vi "Shooter_Motor.vi"(0 "MotorControlDevRef":T2={"DeviceStatus"={"status"=FALSE, "code"=0, "source"=""}, "Type"=enum."PWM", "PWM"={"PWM Channel"=enum."Invalid", "DeadBand"={"Name"="", "maxPositivePwm"=0, "minPositivePwm"=0, "centerPwm"=0, "maxNegativePwm"=0, "minNegativePwm"=0, "angularRange"=0}}, "CAN"={"Device Number"=0, "SetOutput VI Ref"=variant(refnum<vi> refnum), "GetOutput VI Ref"=variant(refnum<vi> refnum), "Enable VI Ref"=variant(refnum<vi> refnum), "Disable VI Ref"=variant(refnum<vi> refnum), "Data"=variant}, "Invert"=FALSE}, 1 "Invert?":bool, 2 "RPM_Input":dbl, 3 "Wanted_RPM":dbl=1.0, 4 "dt_In_PID":dbl, 5 "PID gains":T1={"proportional gain (Kc)"=1.0, "integral time (Ti, min)"=0.01, "derivative time (Td, min)"=0.0} {"derivative time (Td, min)" format="%.3f"; "integral time (Ti, min)" format="%.3f"; "proportional gain (Kc)" format="%.3f"}) -> (14 "Shooter_Speed":dbl, 15 "dt_Out_PID":dbl, 16 "RPM_Reached?":bool)   [LabVIEW 2016]
uses:
  <vilib>/Rock Robotics/WPI/MotorControl/WPI_MotorControlDeviceRef.ctl
  <vilib>/Rock Robotics/WPI/MotorControl/WPI_MotorControlType.ctl
  <vilib>/Rock Robotics/SystemInterfaces/DIO/FPGA_DIOPWMChannel.ctl
  <vilib>/Rock Robotics/WPI/PWM/WPI_PWMDeadband.ctl
  <vilib>/addons/control/pid/pid.llb/PID (DBL).vi
  <vilib>/addons/control/pid/NI_PID_pid.lvlib
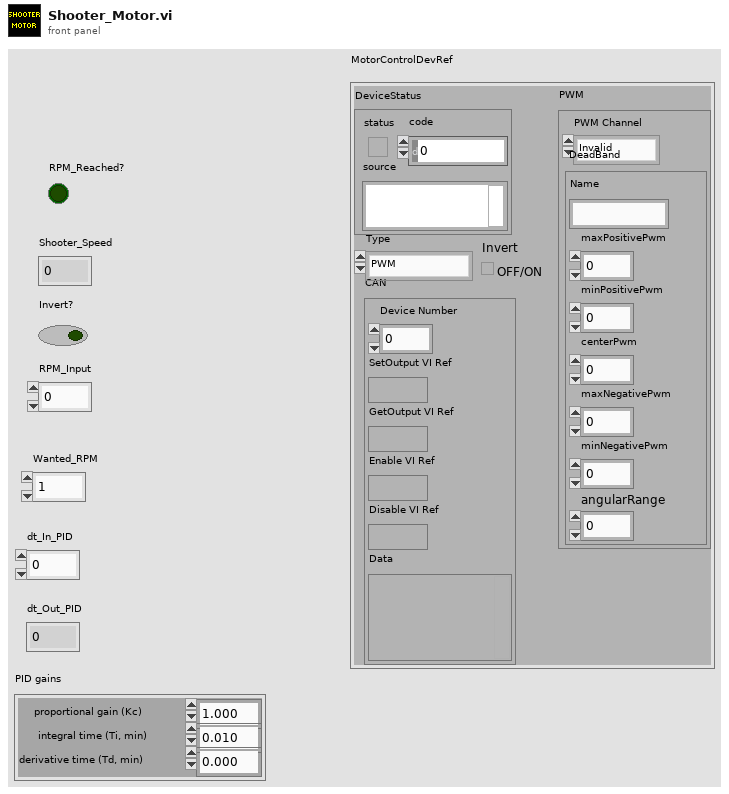
[diagram p1: front panel]
types:
  T1 = cluster{"proportional gain (Kc)":dbl, "integral time (Ti, min)":dbl, "derivative time (Td, min)":dbl}
  T2 = typedef "WPI_MotorControlDeviceRef.ctl" = cluster{"DeviceStatus":errorcluster, "Type":T3, "PWM":cluster{"PWM Channel":T4, "DeadBand":T5}, "CAN":cluster{"Device Number":u8, "SetOutput VI Ref":variant, "GetOutput VI Ref":variant, "Enable VI Ref":variant, "Disable VI Ref":variant, "Data":variant}, "Invert":bool}
  T3 = typedef "WPI_MotorControlType.ctl" = enum16{"PWM", "CAN"}
  T4 = typedef "FPGA_DIOPWMChannel.ctl" = enum8{"PWM 0", "PWM 1", "PWM 2", "PWM 3", "PWM 4", "PWM 5", "PWM 6", "PWM 7", "PWM 8", "PWM 9", "PWM MXP 0", "PWM MXP 1", "PWM MXP 2", "PWM MXP 3", "PWM MXP 4", "PWM MXP 5", "PWM MXP 6", "PWM MXP 7", "PWM MXP 8", "PWM MXP 9", "Invalid"}
  T5 = typedef "WPI_PWMDeadband.ctl" = cluster{"Name":string, "maxPositivePwm":i32, "minPositivePwm":i32, "centerPwm":i32, "maxNegativePwm":i32, "minNegativePwm":i32, "angularRange":u16}
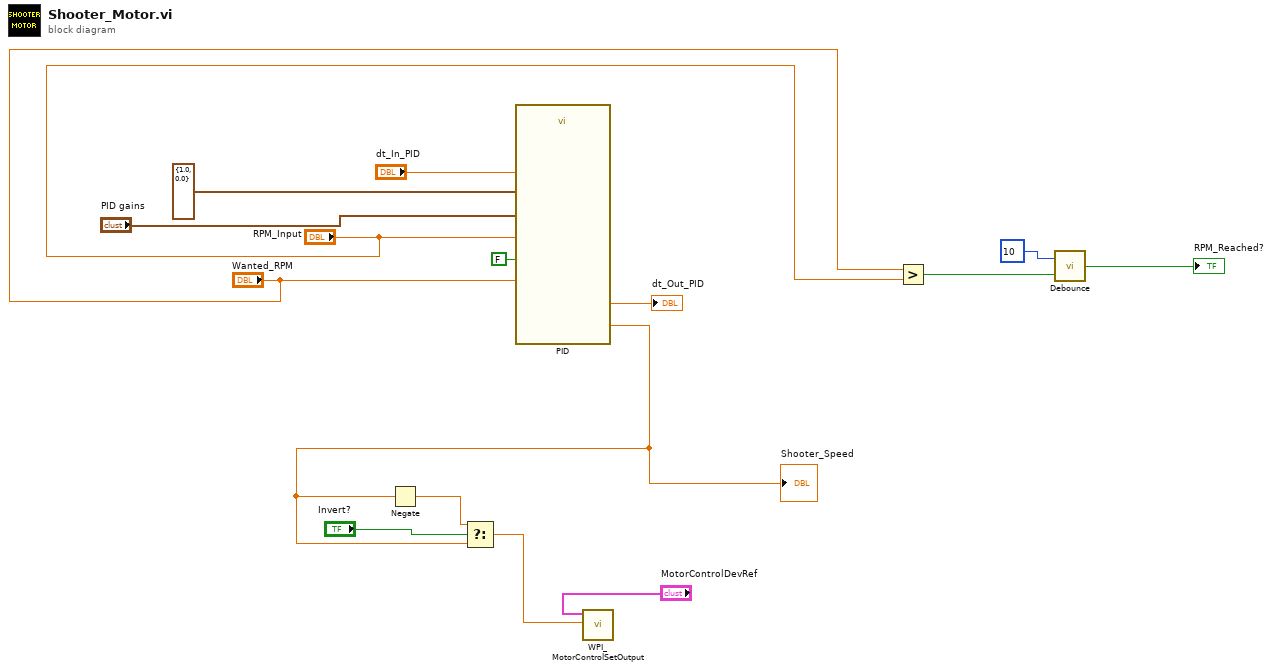
[diagram p0: block diagram]
diagram:
  n1 = call-poly <vilib>:"PID.vi"("reinitialize? (F)"=FALSE, "output range"=cluster{"output high":dbl, "output low":dbl} {"output high"=1.0, "output low"=0.0}, "dt (s)"="dt_In_PID", "PID gains"="PID gains", "process variable"="RPM_Input", "setpoint"="Wanted_RPM") -> ("dt out (s)"=→"dt_Out_PID":dbl, "output"=w9:dbl)  [unwired: 4 in]
  "Shooter_Speed" <- w9
  n2 = Negate(x=w9) -> (-x=w8:dbl)
  n3 = Select(t=w8, s="Invert?", f=w9) -> (s? t:f=w7:dbl)
  n4 = call <vilib>:"WPI_MotorControlSetOutput.vi"("Output"=w7, "MotorControlDevRef"="MotorControlDevRef") -> ()  [unwired: 7 in, 3 out]
  n5 = Greater?(x="Wanted_RPM", y="RPM_Input") -> (0:w3:bool)
  n6 = call "Debounce.vi"("Input"=w3, "Num samples"=10) -> ("Output"=→"RPM_Reached?":bool)
